vi "Unit Delay.vi"   [LabVIEW 2017, in "NI_AdvCtrl_discrete linear.lvlib"]
doc: "LabVIEW no longer supports this VI. You can obtain similar functionality by installing the LabVIEW Simulation Module.\n\nDelays the input exactly one time step, i.e. output point[n]=input point[n-1], where output point[0]=initial condition."
uses:
  <vilib>/addons/control/advanced/NI_AdvCtrl_discrete linear.lvlib
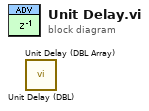
[diagram p0: block diagram]
diagram:
  n1 = call <vilib>:"Unit Delay (DBL).vi"() -> ()  [unwired: 5 in, 1 out]
  n2 = call <vilib>:"Unit Delay (DBL Array).vi"() -> ()  [unwired: 5 in, 1 out]
